vi "Nyquist Plot of a Filter - DFD.vi"() -> ()   [LabVIEW 2023]
doc: "Computes the frequency response function of a digital filter and displays the attenuation versus the frequency, as well as the imaginary part versus the real part (Nyquist plot). This example uses VIs in the LabVIEW Digital Filter Design Toolkit to make the design and plot the response of the filter."
uses:
  <vilib>/addons/Digital Filter Design/Analysis.llb/DFD Plot Freq Response (Linear-Spaced).vi
  <vilib>/addons/Digital Filter Design/Process.llb/DFD Filtering (Wfm).vi
  <vilib>/measure/maspectr.llb/Frequency Response Function (Real-Im) 1-1.vi
  <vilib>/measure/NI_MABase.lvlib
  <vilib>/addons/Digital Filter Design/NI_DigFilterLicensed.lvlib
  <vilib>/measure/NI_MAPro.lvlib
panel:
  in  "Filter specifications":T1={"Topology"=enum."Butterworth", "Type"=enum."Bandpass", "Order"=3, "Lower Fc"=1000.0, "Upper Fc"=2000.0, "PB Ripple"=0.025, "SB Attenuation"=90.0} {"PB Ripple" format="%0.4f"; "Lower Fc" format="%0.2p"; "SB Attenuation" format="%0.2f"; "Upper Fc" format="%0.2p"}
  out "Frequency response":cluster{"f0":dbl, "df":dbl, "values":dbl[]}[](graph)
  out "Nyquist plot":T2(graph)
  in  "stop":bool
  # "Select Help»Show Context Help and move the cursor over the VI icon for more information."
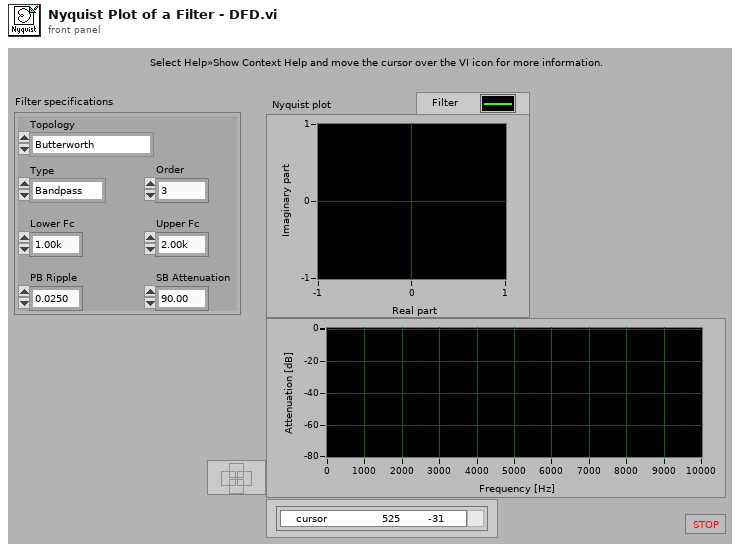
[diagram p1: front panel]
types:
  T1 = cluster{"Topology":enum16{"Off", "Butterworth", "Chebyshev", "Inverse Chebyshev", "Elliptic", "Bessel"}, "Type":enum16{"Lowpass", "Highpass", "Bandpass", "Bandstop"}, "Order":i32, "Lower Fc":dbl, "Upper Fc":dbl, "PB Ripple":dbl, "SB Attenuation":dbl}
  T2 = cluster{"real part":dbl[], "imaginary part":dbl[]}
  T3 = enum16{"None ", "Hanning", "Hamming", "Blackman-Harris", "Exact Blackman", "Blackman", "Flat Top", "4 Term B-Harris ", "7 Term B-Harris", "Low Sidelobe"}
  T4 = cluster{"averaging mode":enum16{"No averaging", "Vector averaging", "RMS averaging"}, "weighting mode":enum16{"Linear", "Exponential"}, "number of averages":u32}
  T5 = typedef "NI_DigFilterLicensed.lvlib/DFD Filter Obj.ctl" = cluster{"mSRate_Fs":dbl, "mSRate_Version":string, "mSRate_Comments":string, "mSRate_OrgCoef":T6, "mSRate_CurCoef":T6, "mSRate_Quantized?":bool, "mSRate_QCoef":T6, "mSRate_QSettings":T8[], "mSRate_Order":i32, "mSRate_Scaling":cluster{"mSRate_ScaleByPowerOf2?":bool, "mSRate_ScaleType":T10}}
  T6 = typedef "NI_DigFilterLicensed.lvlib/DFD Filter Coef.ctl" = cluster{"type":T7, "gain":dbl, "coef a (k)":dbl[], "coef b (v)":dbl[]}
  T7 = typedef "NI_DigFilterLicensed.lvlib/DFD Filter Structure Type Selector.ctl" = enum16{"Undefined", "FIR Direct Form", "FIR Direct Form Transposed", "FIR Symmetric", "FIR Antisymmetric", "IIR Direct Form I", "IIR Direct Form I Transposed", "IIR Direct Form II", "IIR Direct Form II Transposed", "IIR Cascaded Second Order Sections Form I", "IIR Cascaded Second Order Sections Form I Transposed", "IIR Cascaded Second Order Sections Form II", "IIR Cascaded Second Order Sections Form II Transposed", "Lattice Allpass (basic sections)", "Lattice Allpass (one multiplier sections)", "Lattice Allpass (normalized sections)", "Lattice AR (basic sections)", "Lattice AR (one multiplier sections)", "Lattice AR (normalized sections)", "Lattice MA (minimum phase)", "Lattice MA (maximum phase)", "Lattice ARMA (basic sections)", "Lattice ARMA (one multiplier sections)", "Lattice ARMA (normalized sections)"}
  T8 = typedef "NI_DigFilterLicensed.lvlib/dfd_Internal Quantization Settings.ctl" = cluster{"source":T9, "wl":i16, "iwl":i16, "overflow mode":enum16{"Saturation", "Wrap"}, "rounding mode":enum16{"Nearest", "Truncation"}, "signed?":bool}
  T9 = typedef "NI_DigFilterLicensed.lvlib/dfd_Internal Quantization Srcs.ctl" = u16
  T10 = typedef "NI_DigFilterLicensed.lvlib/DFD Coef Norm Type.ctl" = enum16{"No Norm", "Time Domain 1-Norm", "Time Domain 2-Norm", "Time Domain Inf-Norm"}
  T11 = cluster{"f0":dbl, "df":dbl, "imaginary part":dbl[]}
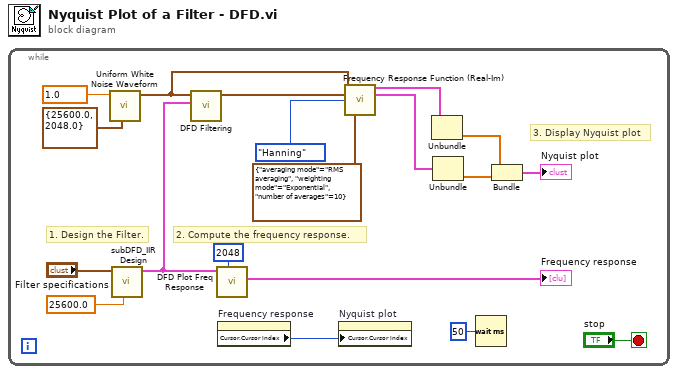
[diagram p0: block diagram]
diagram:
  n1 = while {
    stop <- "stop" stop-if-true
    # "3. Display Nyquist plot"
    # "1. Design the Filter."
    # "2. Compute the frequency response."
    n2 = call <vilib>:"Uniform White Noise Waveform.vi"("sampling info"=cluster{"Fs":dbl, "#s":dbl} {"Fs"=25600.0, "#s"=2048.0}, "amplitude"=1.0 ("Amplitude")) -> ("signal out"=w7:waveform(dbl))  [unwired: 3 in, 6 out]
    n3 = call "subDFD_IIR Design.vi"("fs [Hz]"=25600.0 ("Fs"), "Filter specifications"="Filter specifications") -> ("filter out"=w9:T5)  [unwired: 9 out]
    n4 = call-poly <vilib>:"DFD Filtering.vi"("filter"=w9, "signal in"=w7) -> ("signal out"=w8:waveform(dbl))  [unwired: 2 in, 7 out]
    n5 = call-poly <vilib>:"DFD Plot Freq Response.vi"("# freq bins"=2048 ("# freq bins (auto)"), "filter in"=w9) -> ("magnitude response"=→"Frequency response":cluster{"f0":dbl, "df":dbl, "values":dbl[]}[])  [unwired: 6 in, 3 out]
    n6 = property on="Frequency response" class="WFGraph (strict)"() -> ("Cursor.Cursor Index"=w17:i32)  [unwired: 2 in, 2 out]
    n7 = property on="Nyquist plot" class="XYGraph (strict)"("Cursor.Cursor Index"=w17) -> ()  [unwired: 2 in, 2 out]
    n8 = call-poly <vilib>:"Frequency Response Function (Real-Im).vi"("time signal X"=w7, "time signal Y"=w8, "window"=T3."Hanning", "averaging parameters"=T4 {"averaging mode"=enum."RMS averaging", "weighting mode"=enum."Exponential", "number of averages"=10}) -> ("real part"=w5:cluster{"f0":dbl, "df":dbl, "real part":dbl[]}, "imaginary part"=w4:T11)  [unwired: 3 in, 7 out]
    n9 = Unbundle(w5) -> ("real part"=w3:dbl[])  [unwired: 2 out]
    n10 = Unbundle(w4) -> ("imaginary part"=w2:dbl[])  [unwired: 2 out]
    n11 = Wait (ms)(milliseconds to wait=u32 50) -> ()  [unwired: 1 out]
    n12 = Bundle("real part"=w3, "imaginary part"=w2) -> (→"Nyquist plot":T2)  [unwired: 1 out]
  }
